vi "GetProperties.vi"(8 "error in":errorcluster, 11 "NamedNumeric in":refnum<class "NamedNumeric.lvclass">) -> (0 "error out":errorcluster, 3 "NamedNumeric out":refnum<class "NamedNumeric.lvclass">)   [LabVIEW 2014, in "Raspberry Pi Compatible Compiler for LabVIEW.lvlib" / "NamedNumeric.lvclass"]
uses:
  NamedNumeric.lvclass
  NamedNumeric.lvclass/NamedNumeric.ctl
  Numeric/Numeric.lvclass
  Digital/Digital.lvclass
  Text/Text.lvclass
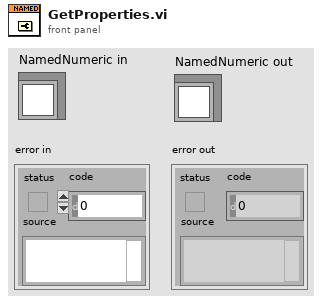
[diagram p1: front panel]
types:
  T1 = typedef "LVBoundsTypeDef.ctl" = cluster{"Width":u32, "Height":u32}
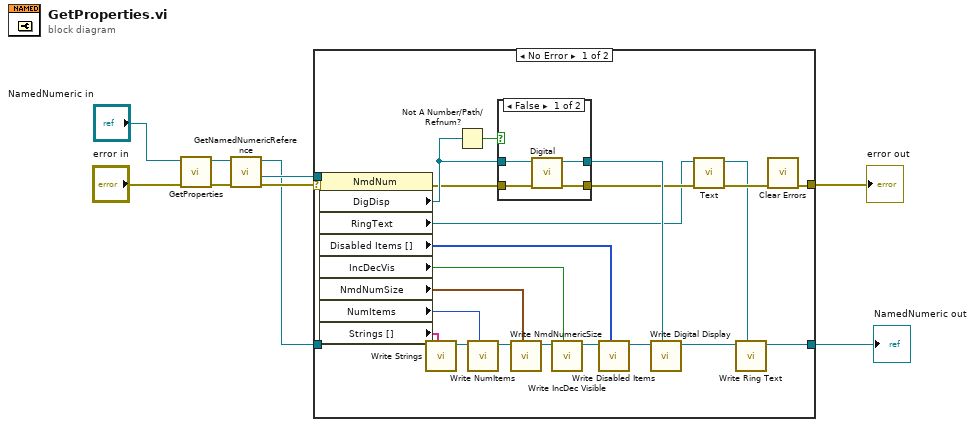
[diagram p0: block diagram]
diagram:
  n1 = call-parent "GetProperties.vi"("error in"="error in", "Numeric in"="NamedNumeric in") -> ("error out"=w3:errorcluster, "Numeric out"=w4:refnum<class "NamedNumeric.lvclass">)  [unwired: 8 in]
  n2 = call "GetNamedNumericReference.vi"("error in"=w3, "NamedNumeric in"=w4) -> ("error out"=w8:errorcluster, "Named Numeric reference"=w7:refnum<vi>, "NamedNumeric out"=w6:refnum<class "NamedNumeric.lvclass">)  [unwired: 7 in]
  n3 = case shown="No Error" w8 {
    selector: w8 -> [w33 w40]
    tunnel: [w10 w40] -> w9
    tunnel: w7 -> [w32 _]
    tunnel: w6 -> [w11 w39]
    tunnel: [w12 w39] -> w5
    frame No Error {
      n4 = property class="NmdNum"(reference=w32, error in=w33) -> (error out=w20:errorcluster, "DigDisp"=w21:refnum<vi>, "RingText"=w16:refnum<vi>, "Disabled Items []"=w23:i32[], "IncDecVis"=w25:bool, "NmdNumSize"=w27:T1, "NumItems"=w29:u32, "Strings []"=w31:string[])  [unwired: 1 out]
      n5 = call "Write Strings.vi"("Strings"=w31, "NamedNumeric in"=w11) -> ("NamedNumeric out"=w30:refnum<class "NamedNumeric.lvclass">)  [unwired: 7 in]
      n6 = Not A Number/Path/Refnum?(number/path/refnum=w21) -> (NaN/Path/Refnum?=w22:bool)
      n7 = call "Write NumItems.vi"("NumItems"=w29, "NamedNumeric in"=w30) -> ("NamedNumeric out"=w28:refnum<class "NamedNumeric.lvclass">)  [unwired: 7 in]
      n8 = case shown="False" w22 {
        tunnel: w21 -> [w36 _]
        tunnel: w20 -> [w37 w38]
        tunnel: [w35 _] -> w19
        tunnel: [w34 w38] -> w17
        frame False {
          n9 = call "Digital.vi"("error in"=w37, "GObj Refnum"=w36) -> ("error out"=w34:errorcluster, "Digital out"=w35:refnum<class "Digital.lvclass">)  [unwired: 8 in]
        }
        frame True {
        }
      }
      n10 = call "Write NmdNumericSize.vi"("NmdNumericSize"=w27, "NamedNumeric in"=w28) -> ("NamedNumeric out"=w26:refnum<class "NamedNumeric.lvclass">)  [unwired: 7 in]
      n11 = call "Write IncDec Visible.vi"("IncDec Visible"=w25, "NamedNumeric in"=w26) -> ("NamedNumeric out"=w24:refnum<class "NamedNumeric.lvclass">)  [unwired: 7 in]
      n12 = call "Write Disabled Items.vi"("Disabled Items"=w23, "NamedNumeric in"=w24) -> ("NamedNumeric out"=w18:refnum<class "NamedNumeric.lvclass">)  [unwired: 7 in]
      n13 = call "Write Digital Display.vi"("Digital Display"=w19, "NamedNumeric in"=w18) -> ("NamedNumeric out"=w14:refnum<class "NamedNumeric.lvclass">)  [unwired: 7 in]
      n14 = call "Text.vi"("error in"=w17, "Gen Refnum"=w16) -> ("error out"=w15:errorcluster, "Text out"=w13:refnum<class "Text.lvclass">)  [unwired: 8 in]
      n15 = call "Write Ring Text.vi"("Ring Text"=w13, "NamedNumeric in"=w14) -> ("NamedNumeric out"=w12:refnum<class "NamedNumeric.lvclass">)  [unwired: 7 in]
      n16 = call <vilib>:"Clear Errors.vi"("error in (no error)"=w15) -> ("error out"=w10:errorcluster)  [unwired: 5 in, 1 out]
    }
    frame Error {
    }
  }
  "error out" <- w9
  "NamedNumeric out" <- w5
